vi "Initialize.vi"(8 "error in":errorcluster, 9 "Number of Channels":u32=1, 10 "Plugin Name":string, 11 "Power Limits in":refnum<class "Power Limits.lvclass">) -> (0 "error out":errorcluster, 3 "Power Limits out":refnum<class "Power Limits.lvclass">)   [LabVIEW 2023, in "Power Limits.lvclass"]
uses:
  Power Limits.lvclass
  Power Limits.lvclass/Power Limits.ctl
  <vilib>/ADAS Replay HIL/Channels/Tag Wrapper/Polymorphic/Open Consumer Tag (Double).vi
  <vilib>/ADAS Replay HIL/Channels/Tag Wrapper/Polymorphic/Set Default Value (Double).vi
  <vilib>/ADAS Replay HIL/Channels/Tag Wrapper/Polymorphic/Open Consumer Tag (Double).vi/bacb721e-673a-491a-accd-959f2e1f334e.vi
  <vilib>/ADAS Replay HIL/Channels/Tag Wrapper/Polymorphic/Set Default Value (Double).vi/228e99de-6fcf-414d-86fc-dc277c7b351f.vi
  <vilib>/ADAS Replay HIL/Channels/Tag Wrapper/Polymorphic/Open Consumer Tag (Double).vi/bacb721e-673a-491a-accd-959f2e1f334e.vi/c28b0ead-42ad-4072-80a2-aca7f2bd7ce3.vi
  <vilib>/ADAS Replay HIL/Channels/Tag Wrapper/Polymorphic/Set Default Value (Double).vi/228e99de-6fcf-414d-86fc-dc277c7b351f.vi/4bc1c15b-36ab-481f-b8dd-c64075ce723a.vi
  <vilib>/ADAS Replay HIL/AdasHilServices/AdasHilServices Fill In Error Info Ex.vi
  <vilib>/ADAS Replay HIL/Channels/Tag Wrapper/Tag Wrapper.lvlib
  Utilities/Utilities.lvlib
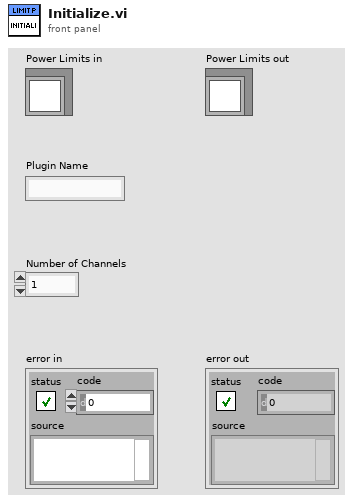
[diagram p1: front panel]
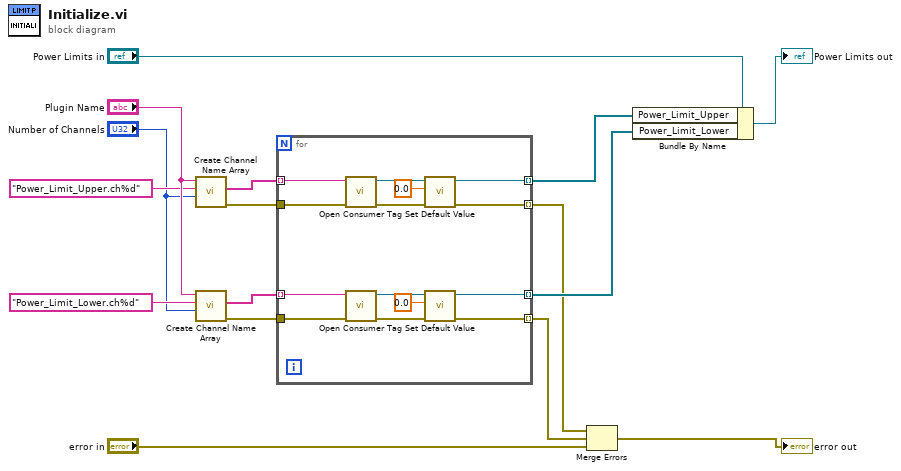
[diagram p0: block diagram]
diagram:
  n1 = call "Create Channel Name Array.vi"("Number of Channels"="Number of Channels", "Channel Format String"="Power_Limit_Upper.ch%d" ("Channel Name"), "Plugin Name"="Plugin Name") -> ("error out"=w1:errorcluster, "Channel Names"=w4:string[])  [unwired: 7 in]
  n2 = call "Create Channel Name Array.vi"("Number of Channels"="Number of Channels", "Channel Format String"="Power_Limit_Lower.ch%d" ("Channel Name"), "Plugin Name"="Plugin Name") -> ("error out"=w2:errorcluster, "Channel Names"=w3:string[])  [unwired: 7 in]
  n3 = for {
    tunnel: [w26] -> w14 mode=indexing
    tunnel: [w25] -> w13 mode=indexing
    tunnel: [w24] -> w12 mode=indexing
    tunnel: [w23] -> w11 mode=indexing
    tunnel: w4 -> [w20] mode=indexing
    tunnel: w3 -> [w19] mode=indexing
    tunnel: w2 -> [w18]
    tunnel: w1 -> [w17]
    n4 = call-poly <vilib>:"Open Consumer Tag.vi"("error in"=w17, "Channel Name"=w20) -> ("error out"=w29:errorcluster, "ADAS HIL Channel"=w30:refnum<k21>)  [unwired: 8 in]
    n5 = call-poly <vilib>:"Open Consumer Tag.vi"("error in"=w18, "Channel Name"=w19) -> ("error out"=w27:errorcluster, "ADAS HIL Channel"=w28:refnum<k21>)  [unwired: 8 in]
    n6 = call-poly <vilib>:"Set Default Value.vi"("error in"=w29, "Default Value"=0.0, "ADAS HIL Channel in"=w30) -> ("error out"=w24:errorcluster, "ADAS HIL Channel out"=w26:refnum<k21>)  [unwired: 7 in]
    n7 = call-poly <vilib>:"Set Default Value.vi"("error in"=w27, "Default Value"=0.0, "ADAS HIL Channel in"=w28) -> ("error out"=w23:errorcluster, "ADAS HIL Channel out"=w25:refnum<k21>)  [unwired: 7 in]
  }
  n8 = Merge Errors(w12, w11, "error in") -> (→"error out":errorcluster)
  n9 = Bundle By Name(cluster="Power Limits in", "Power_Limit_Upper"=w14, "Power_Limit_Lower"=w13) -> (→"Power Limits out":refnum<class "Power Limits.lvclass">)
